vi "OnDoubleClickRuntime2.vi"(0 "XRef":T7, 1 "Point":T5, 2 "Mouse Mods":T3, 3 "State In":T2) -> (14 "Fatal Error Out":T1)   [LabVIEW 2022 SP3, in "Flex Block.xnode"]
uses:
  Flex Block.xnode
  <vilib>/XNodeSupport/XNodeXNodeRef.ctl
  <vilib>/XNodeSupport/XNodePoint.ctl
  <vilib>/XNodeSupport/XNodeInt.ctl
  <vilib>/XNodeSupport/XNodeMouseMods.ctl
  <vilib>/XNodeSupport/XNodeBool.ctl
  State.ctl
  <vilib>/XNodeSupport/XNodeErrorCluster.ctl
  <vilib>/XNodeSupport/NI_XNodeSupport.lvlib
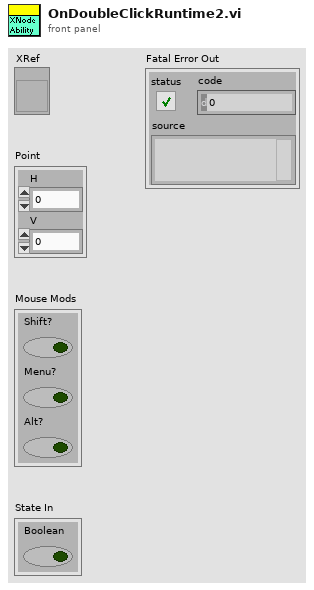
[diagram p1: front panel]
types:
  T1 = typedef "NI_XNodeSupport.lvlib/XNodeErrorCluster.ctl" = errorcluster
  T2 = typedef "Flex Block.xnode/State.ctl" = cluster{"Boolean":bool}
  T3 = typedef "NI_XNodeSupport.lvlib/XNodeMouseMods.ctl" = cluster{"Shift?":T4, "Menu?":T4, "Alt?":T4}
  T4 = typedef "NI_XNodeSupport.lvlib/XNodeBool.ctl" = bool
  T5 = typedef "NI_XNodeSupport.lvlib/XNodePoint.ctl" = cluster{"H":T6, "V":T6}
  T6 = typedef "NI_XNodeSupport.lvlib/XNodeInt.ctl" = i32
  T7 = typedef "NI_XNodeSupport.lvlib/XNodeXNodeRef.ctl" = refnum<vi>
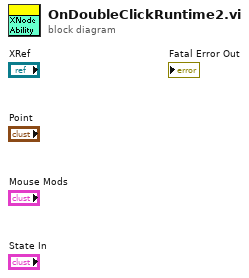
[diagram p0: block diagram]
diagram:
